vi "Create Dialog (by ref).vi"(5 "Bar Visibility":T2={"Menu Bar"=FALSE, "Title Bar"=TRUE}, 6 "Calling VI Reference":refnum<vi>, 7 "Scrollbars (off)":T3, 8 "error in":errorcluster, 9 "Launch Position (Centered)":T1=enum."Centered", 10 "Dialog Behavior":T4(ring)=enum."Default", 11 "UI VI Reference (caller)":refnum<vi>) -> (0 "error out":errorcluster, 3 "Philips Dialog out":refnum<class "Flex UI Dialog.lvclass">)   [LabVIEW 2014, in "Flex UI Dialog.lvclass"]
doc: "Generates a Dialog with all the associated behavior from the input UI VI Reference.\n\nIf no reference is given, uses the calling VI."
uses:
  Flex UI Dialog.lvclass
  Cluster - Scrollbar Settings.ctl
  Cluster - Bar Visibility.ctl
  Enum - Launch Position.ctl
  Flex UI (Parent)/Flex UI.lvclass/Flex UI.ctl
  Flex UI Dialog.lvclass/Flex UI Dialog.ctl
  Flex UI (Parent)/Flex UI.lvclass
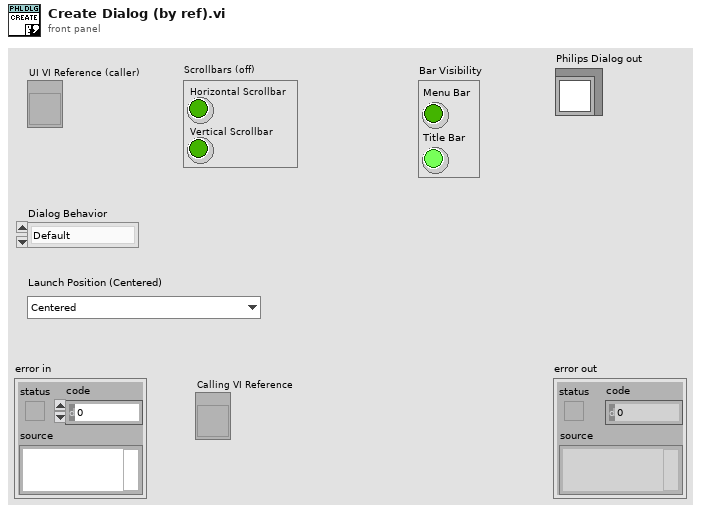
[diagram p1: front panel]
types:
  T1 = typedef "Flex UI Dialog.lvclass/Enum - Launch Position.ctl" = enum16{"Default (Last Opened)", "Centered", "Centered on Caller", "Maximized", "Hidden"}
  T2 = typedef "Flex UI Dialog.lvclass/Cluster - Bar Visibility.ctl" = cluster{"Menu Bar":bool, "Title Bar":bool}
  T3 = typedef "Flex UI Dialog.lvclass/Cluster - Scrollbar Settings.ctl" = cluster{"Horizontal Scrollbar":bool, "Vertical Scrollbar":bool}
  T4 = enum32{"Invalid", "Default", "Floating", "Floating/Auto-Hide", "Modal"}
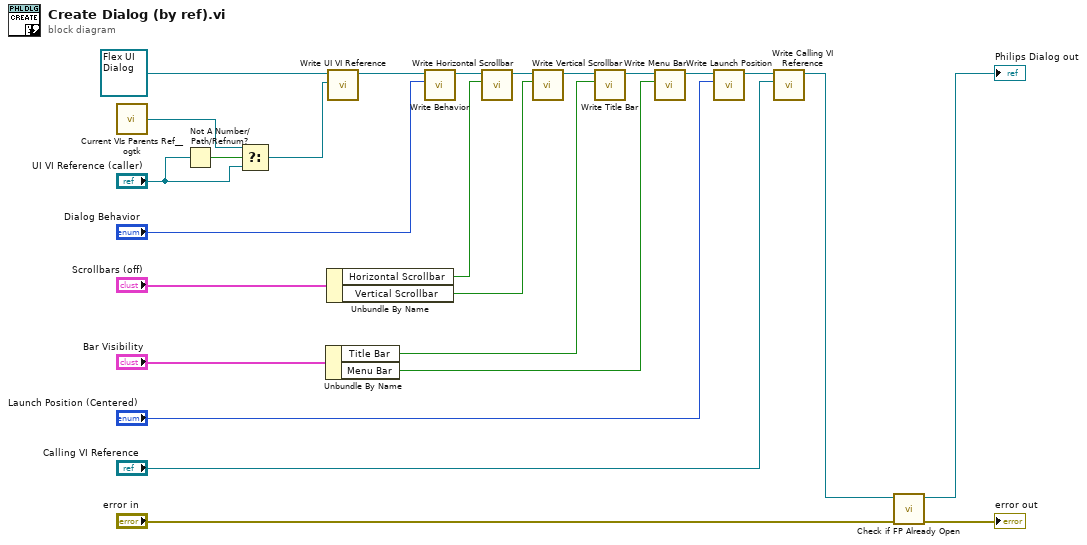
[diagram p0: block diagram]
diagram:
  n1 = call <userlib>:"Current VIs Parents Ref__ogtk.vi"() -> ("Calling VI's Reference"=w20:refnum<vi>)  [unwired: 2 in]
  n2 = Not A Number/Path/Refnum?(number/path/refnum="UI VI Reference (caller)") -> (NaN/Path/Refnum?=w21:bool)
  n3 = Select(t=w20, s=w21, f="UI VI Reference (caller)") -> (s? t:f=w18:refnum<vi>)
  n4 = Unbundle By Name("Bar Visibility") -> ("Title Bar"=w8:bool, "Menu Bar"=w7:bool)
  n5 = Unbundle By Name("Scrollbars (off)") -> ("Horizontal Scrollbar"=w11:bool, "Vertical Scrollbar"=w10:bool)
  n6 = call "Write UI VI Reference.vi"("UI VI Reference"=w18, "Philips UI in"=refnum<class "Flex UI Dialog.lvclass"> refnum ("Philips Dialog out")) -> ("Philips UI out"=w23:refnum<class "Flex UI Dialog.lvclass">)  [unwired: 9 in]
  n7 = call "Write Behavior.vi"("Behavior"="Dialog Behavior", "Philips Dialog in"=w23) -> ("Philips Dialog out"=w13:refnum<class "Flex UI Dialog.lvclass">)  [unwired: 9 in]
  n8 = call "Write Horizontal Scrollbar.vi"("Horizontal Scrollbar"=w11, "Philips Dialog in"=w13) -> ("Philips Dialog out"=w17:refnum<class "Flex UI Dialog.lvclass">)  [unwired: 9 in]
  n9 = call "Write Vertical Scrollbar.vi"("Vertical Scrollbar"=w10, "Philips Dialog in"=w17) -> ("Philips Dialog out"=w16:refnum<class "Flex UI Dialog.lvclass">)  [unwired: 9 in]
  n10 = call "Write Title Bar.vi"("Title Bar"=w8, "Philips Dialog in"=w16) -> ("Philips Dialog out"=w15:refnum<class "Flex UI Dialog.lvclass">)  [unwired: 9 in]
  n11 = call "Write Menu Bar.vi"("Menu Bar"=w7, "Philips Dialog in"=w15) -> ("Philips Dialog out"=w14:refnum<class "Flex UI Dialog.lvclass">)  [unwired: 9 in]
  n12 = call "Write Launch Position.vi"("Launch Position"="Launch Position (Centered)", "Philips Dialog in"=w14) -> ("Philips Dialog out"=w4:refnum<class "Flex UI Dialog.lvclass">)  [unwired: 9 in]
  n13 = call "Write Calling VI Reference.vi"("Calling VI Reference"="Calling VI Reference", "Philips Dialog in"=w4) -> ("Philips Dialog out"=w2:refnum<class "Flex UI Dialog.lvclass">)  [unwired: 9 in]
  n14 = call "Check if FP Already Open.vi"("error in"="error in", "Philips Dialog in"=w2) -> ("error out"=→"error out":errorcluster, "Philips Dialog out"=→"Philips Dialog out":refnum<class "Flex UI Dialog.lvclass">)  [unwired: 8 in]
